vi "SC_schleife.vi"   [LabVIEW 2016]
uses:
  Oxford Software/Oxsoft/RAMP.LLB/RampTState.ctl
  Global/Global Variables/global.vi
  Global/Global Variables/Data_Display_global.vi
  CryoTUM-V1.0/Instrument_Setup.vi
types:
  T1 = typedef "RampTState.ctl" = enum16{"START", "RUN"}
  T2 = typedef "PSIO.ctl" = cluster{"Address":T3, "Version":enum16{"PS", "IPS"}}
  T3 = typedef "OxfordAddress.ctl" = cluster{"Com Port":i32, "ISOBUS Address":i32, "GPIB Address":i16, "Communication":enum16{"RS232", "ISOBUS", "GPIB", "Gateway"}}
  T4 = cluster{"ControlTITC":i8, "ControlTCh":i8, "SampleTITC":i8, "SampleTCh":i8}
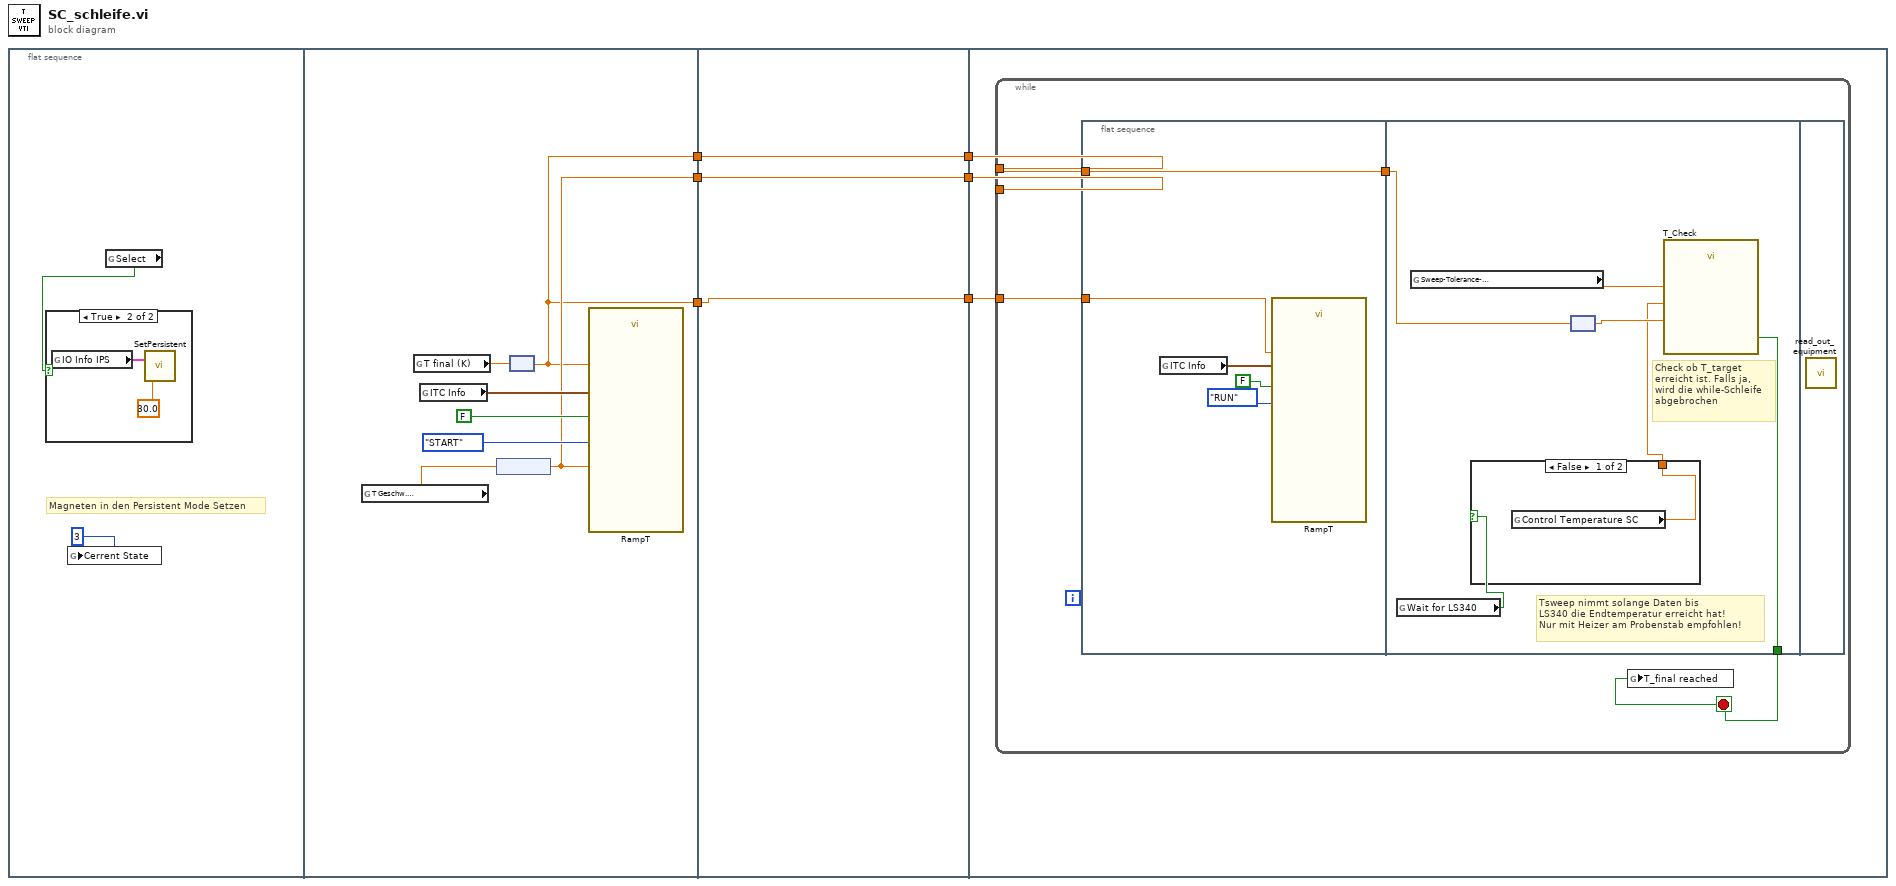
[diagram p0: block diagram]
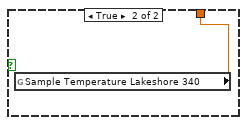
[diagram p3: hidden frame]
diagram:
  n1 = flat-sequence {
    tunnel: [w12] -> w4
    tunnel: [w11] -> w6
    tunnel: [w11] -> w2
    tunnel: w6 -> [w20]
    tunnel: [w20] -> w5
    tunnel: w4 -> [w19]
    tunnel: [w19] -> w3
    tunnel: w2 -> [w18]
    tunnel: [w18] -> w1
    tunnel: w5 -> [w22]
    tunnel: w3 -> [w23]
    tunnel: w1 -> [w21]
    frame #0 {
      # "Magneten in den Persistent Mode Setzen"
      n2 = global write "global.vi" "Cerrent State"(3) -> ()
      n3 = global read "Data_Display_global.vi" "Select"() -> (w8:bool)
      n4 = case shown="True" w8 {
        frame False {
        }
        frame True {
          n5 = global read "Instrument_Setup.vi" "IO Info IPS"() -> (w9:T2)
          n6 = call "SetPersistent.vi"("Switch Heater Dwell Time"=dbl[unit] 30.0, "IO Info"=w9) -> ()  [unwired: 1 in, 1 out]
        }
      }
    }
    frame #1 {
      n7 = global read "global.vi" "T Geschw. \n(K/min)"() -> (w17:dbl)
      n8 = global read "global.vi" "T final (K)"() -> (w16:dbl)
      n9 = global read "Instrument_Setup.vi" "ITC Info"() -> (w13:T4)
      n10 = node(w17) -> (w12:dbl[unit])
      n11 = node(w16) -> (w11:dbl[unit])
      n12 = call "RampT.vi"("ITC Info"=w13, "Rate"=w12, "Final Temperature"=w11, "JustReadTemperature"=FALSE, "RampTState"=RampTState."START") -> ()  [unwired: 5 out]
    }
    frame #2 {
    }
    frame #3 {
      n13 = while {
        tunnel: w23 -> [_]
        tunnel: w22 -> [w27]
        tunnel: w21 -> [w24]
        stop <- w26 stop-if-true
        n14 = flat-sequence {
          tunnel: w27 -> [w32]
          tunnel: [w32] -> w25
          tunnel: w24 -> [w28]
          tunnel: [w36] -> w26
          tunnel: w25 -> [w38]
          frame #0 {
            n15 = global read "Instrument_Setup.vi" "ITC Info"() -> (w31:T4)
            n16 = call "RampT.vi"("ITC Info"=w31, "Final Temperature"=w28, "JustReadTemperature"=FALSE, "RampTState"=RampTState."RUN") -> ()  [unwired: 1 in, 5 out]
          }
          frame #1 {
            # "Tsweep nimmt solange Daten bis \nLS340 die Endtemperatur erreicht hat!\nNur mit Heizer am Probenstab empfohlen!"
            # "Check ob T_target\nerreicht ist. Falls ja,\nwird die while-Schleife\nabgebrochen"
            n17 = global read "Instrument_Setup.vi" "Wait for LS340"() -> (w33:bool)
            n18 = global read "Instrument_Setup.vi" "Sweep-Tolerance-\nTemperature"() -> (w35:dbl)
            n19 = case shown="False" w33 {
              tunnel: [w39 w40] -> w34
              frame False {
                n20 = global read "Data_Display_global.vi" "Control Temperature SC"() -> (w39:dbl)
              }
              frame True {
                n21 = global read "Data_Display_global.vi" "Sample Temperature Lakeshore 340"() -> (w40:dbl)
              }
            }
            n22 = node(w38) -> (w37:dbl)
            n23 = call "T_Check.vi"("Sweep\nTolerance %"=w35, "T_target (K)"=w37, "T_in"=w34) -> ("= T target"=w36:bool)
          }
          frame #2 {
            n24 = call "read_out_equipment.vi"() -> ()  [unwired: 1 in]
          }
        }
        n25 = global write "Data_Display_global.vi" "T_final reached"(w26) -> ()
      }
    }
  }
